vi "Main.vi"(8 "Error In":errorcluster) -> (0 "Error Out":errorcluster)   [LabVIEW 2017, in "UserInterface.lvlib"]
uses:
  UserInterface.lvlib
  InternalData.ctl
  UserEvents/StopUE.lvlib
  ErrorHandler/ErrorHandler.lvlib
  Controller/Controller.lvlib
panel:
  out "Reply Data":dbl
  in  "WaitOnReply":bool
  in  "DoSomething":bool
  in  "STOP":bool
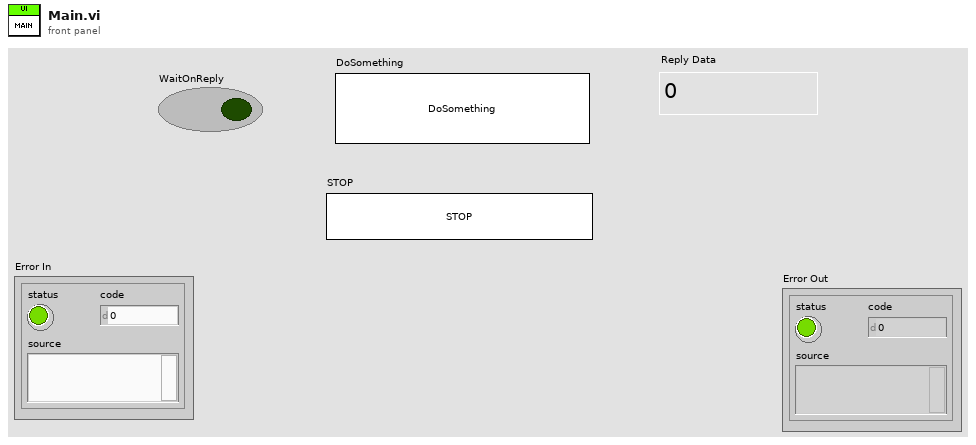
[diagram p1: front panel]
types:
  T1 = typedef "UserInterface.lvlib/InternalData.ctl" = cluster{"Status":string}
  T2 = typedef "UserInterface.lvlib/States_Module.ctl" = enum16{"DoSomething", "Shutdown", "Initialize"}
  T3 = typedef "UserInterface.lvlib/MessageData.ctl" = cluster{"State":T2, "Payload":variant, "WaitOnReply":bool, "ReplyNotif":refnum<notifier>}
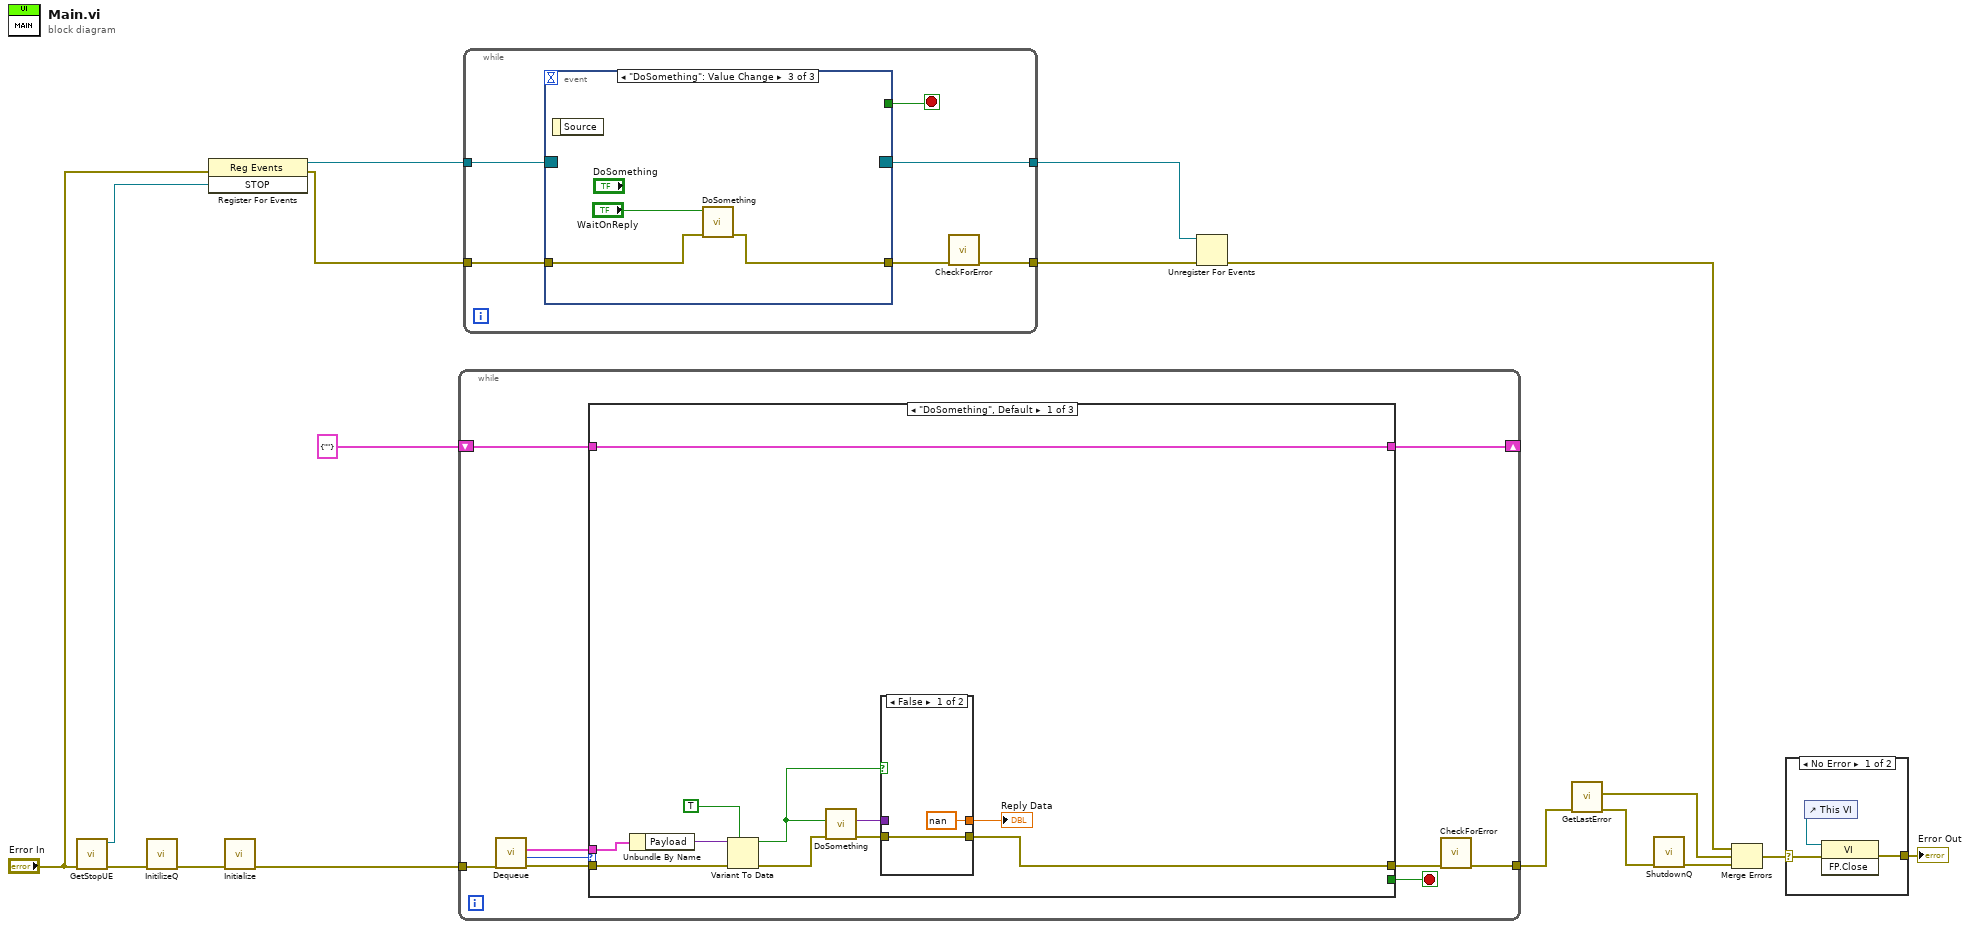
[diagram p0: block diagram]
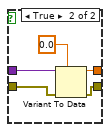
[diagram p3: hidden frame]
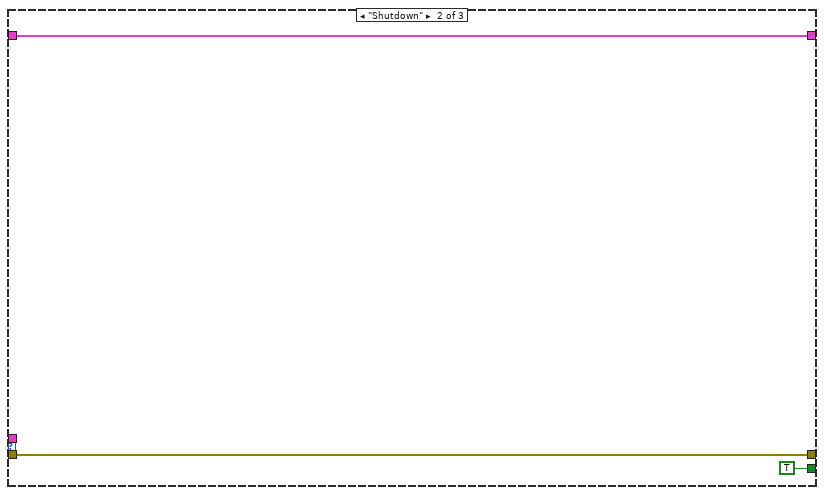
[diagram p4: hidden frame]
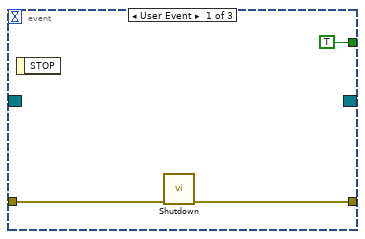
[diagram p6: hidden frame]
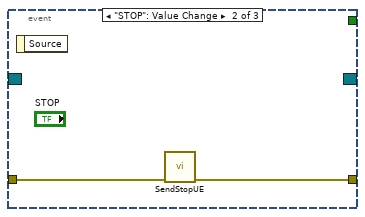
[diagram p7: hidden frame]
diagram:
  n1 = call "GetStopUE.vi"("Error In"="Error In") -> ("Error Out"=w14:errorcluster, "STOP"=w17:refnum<user-event>)  [unwired: 9 in]
  n2 = call "InitilizeQ.vi"("Error In"=w14) -> ("Error Out"=w12:errorcluster)  [unwired: 10 in]
  n3 = register-events(error in="Error In", w17) -> (reference out=w16:refnum<event-registration>, error out=w15:errorcluster)  [unwired: 1 in]
  n4 = call "Initialize.vi"("Error In"=w12) -> ("error out"=w11:errorcluster)  [unwired: 9 in, 1 out]
  n5 = while {
    tunnel: w11 -> [w26]
    tunnel: [w19] -> w8
    shift-right: [w21] -> _
    shift-left: T1 {"Status"=""} ("InternalData") -> [w22]
    stop <- w23 stop-if-true
    n6 = call "Dequeue.vi"("Error In"=w26) -> ("error out"=w25:errorcluster, "State"=w24:T2, "Data out"=w18:T3)  [unwired: 8 in]
    n7 = case shown="\"DoSomething\", Default" w24 {
      tunnel: w25 -> [w32 w46 w49]
      tunnel: [_ TRUE _] -> w23
      tunnel: [w28 w46 w49] -> w20
      tunnel: w22 -> [w37 w45 w48]
      tunnel: [w37 w45 w48] -> w21
      tunnel: w18 -> [w33 _ _]
      frame "DoSomething", Default {
        n8 = Unbundle By Name(w33) -> ("Payload"=w31:variant)
        n9 = Variant To Data(error in=w32, type=TRUE, Variant=w31) -> (data=w27:bool, error out=w29:errorcluster)
        n10 = call "DoSomething.vi"("Error In"=w29, "WaitOnReply"=w27) -> ("error out"=w36:errorcluster, "Reply"=w35:variant)  [unwired: 8 in]
        n11 = case shown="False" w27 {
          tunnel: w36 -> [w39 w43]
          tunnel: w35 -> [_ w44]
          tunnel: [w39 w41] -> w28
          tunnel: [nan ("Reply Data") w40] -> w34
          frame False {
          }
          frame True {
            n12 = Variant To Data(error in=w43, type=0.0 ("Reply Data"), Variant=w44) -> (data=w40:dbl, error out=w41:errorcluster)
          }
        }
        "Reply Data" <- w34
      }
      frame "Shutdown" {
      }
      frame "Initialize" {
      }
    }
    n13 = call "CheckForError.vi"("Error In"=w20) -> ("error out"=w19:errorcluster)  [unwired: 10 in]
  }
  n14 = while {
    tunnel: w16 -> [w55]
    tunnel: w15 -> [w53]
    tunnel: [w50] -> w10
    tunnel: [w52] -> w9
    stop <- w54 stop-if-true
    n15 = event shown="[2] \"DoSomething\": Value Change" {
      selector: w55 -> [_ _ _]
      dyn-events: [_ _ _] -> w52
      timeout: _ -> [_ _ _]
      tunnel: [TRUE _ _] -> w54
      tunnel: w53 -> [w57 w60 w63]
      tunnel: [w56 w59 w61] -> w51
      event User Event {
        n16 = event-data() -> ()  [unwired: 1 in, 1 out]
        n17 = call "Shutdown.vi"("Error In"=w57) -> ("error out"=w56:errorcluster)  [unwired: 9 in, 1 out]
      }
      event "STOP": Value Change {
        n18 = event-data() -> ()  [unwired: 1 in, 1 out]
        n19 = call "SendStopUE.vi"("Error In"=w60) -> ("Error Out"=w59:errorcluster)  [unwired: 10 in]
      }
      event "DoSomething": Value Change {
        n20 = event-data() -> ()  [unwired: 1 in, 1 out]
        n21 = call "DoSomething.vi"("Error In"=w63, "Payload"="WaitOnReply") -> ("error out"=w61:errorcluster)  [unwired: 8 in, 1 out]
      }
    }
    n22 = call "CheckForError.vi"("Error In"=w51) -> ("error out"=w50:errorcluster)  [unwired: 10 in]
  }
  n23 = Unregister For Events(event registration refnum=w9, error in=w10) -> (error out=w4:errorcluster)
  n24 = call "GetLastError.vi"("Error In"=w8) -> ("error IO"=w7:errorcluster, "Last Error"=w5:errorcluster)  [unwired: 9 in]
  n25 = call "ShutdownQ.vi"("Error In"=w7) -> ("Error Out"=w6:errorcluster)  [unwired: 10 in]
  n26 = Merge Errors(w4, w5, w6) -> (w1:errorcluster)
  n27 = case shown="No Error" w1 {
    selector: w1 -> [w66 w67]
    tunnel: [w65 w67] -> w2
    frame No Error {
      n28 = control-ref of="This VI"() -> (w64:refnum<vi>)
      n29 = invoke class="VI" method="FP.Close"(reference=w64, error in=w66) -> (error out=w65:errorcluster)  [unwired: 1 in, 2 out]
    }
    frame Error {
    }
  }
  "Error Out" <- w2
